vi "Read Project Path.vi"(8 "error in (no error)":errorcluster, 11 "Session in":refnum<class "Plugin Session.lvclass">) -> (0 "error out":errorcluster, 2 "Project Path":path, 3 "Session out":refnum<class "Plugin Session.lvclass">)   [LabVIEW 2023, in "InstrumentStudio Plugin SDK.lvlib" / "Plugin Session.lvclass"]
doc: "Call this VI to retrieve the absolute path of the InstrumentStudio project file on disk"
uses:
  Plugin Session.lvclass
  Plugin Session.lvclass/Plugin Session.ctl
  Read Session Id.vi
  NationalInstruments.VIHost.Interop.dll
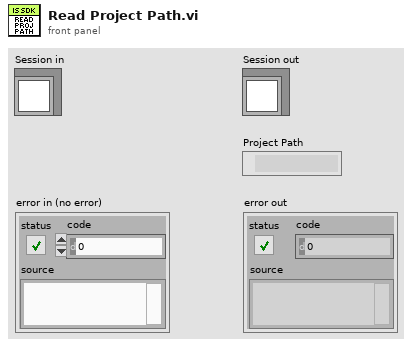
[diagram p1: front panel]
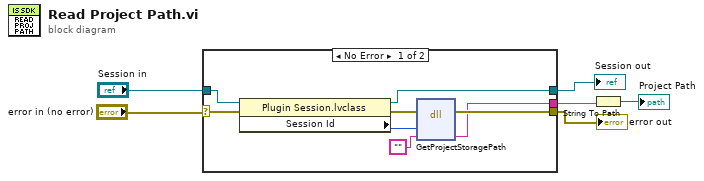
[diagram p0: block diagram]
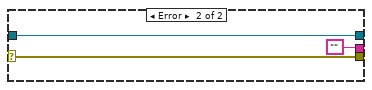
[diagram p2: hidden frame]
diagram:
  n1 = case shown="No Error" "error in (no error)" {
    selector: "error in (no error)" -> [w9 w16]
    tunnel: [w11 w16] -> w6
    tunnel: "Session in" -> [w10 w17]
    tunnel: [w8 w17] -> w3
    tunnel: [w7 ""] -> w2
    frame No Error {
      n2 = property class="Plugin Session.lvclass"(reference=w10, error in=w9) -> (reference out=w8:refnum<class "Plugin Session.lvclass">, error out=w14:errorcluster, "Session Id"=w13:u64)
      n3 = dll-call lib="C:/Users/nmurphy/Downloads/InstrumentStudio_LabVIEW_Plugins/LabVIEW/ExampleProject/PluginSDK/NationalInstruments.VIHost.Interop.dll" fn="GetProjectStoragePath"(error in=w14, "hostId"=w13, "projectPath"="") -> (error out=w11:errorcluster, "projectPath"=w7:string)  [unwired: 4 in, 1 out]
    }
    frame Error {
    }
  }
  "error out" <- w6
  "Session out" <- w3
  n4 = String To Path(string=w2) -> (path=→"Project Path":path)
